vi "test-discretization-12-callback.vi"(9 "Y":T1, 10 "T":dbl, 11 "Variant":variant) -> (0 "Error":bool, 3 "output matrix":T1)   [LabVIEW 2019]
uses:
  <vilib>/Analysis/Matrix/Datatypes/RealMatrix.ctl
  <vilib>/Rock Robotics/WPI/ThirdParty/JAS_Junk/TrajLib/MatBuilder_Create.vi
  <vilib>/Rock Robotics/WPI/ThirdParty/JAS_Junk/TrajLib/Trajectory_Library.lvlib
  <vilib>/Analysis/Matrix/NI_Matrix.lvlib
  <vilib>/Analysis/Matrix/Numeric/Multiply/Multiply - RM,R.vi
  <vilib>/Analysis/NI_AALBase.lvlib
  <vilib>/Analysis/baseanly.llb/Real A x B.vi
panel:
  in  "Cluster":cluster{"ContQ":T1, "ContA":T1}
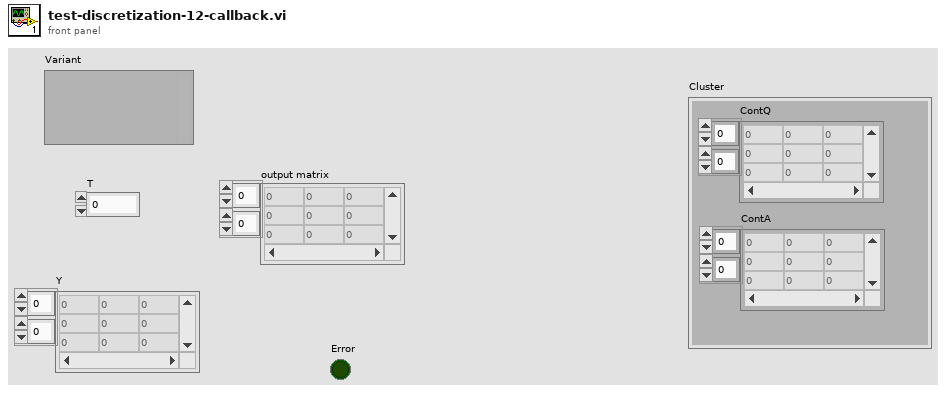
[diagram p1: front panel]
types:
  T1 = typedef "NI_Matrix.lvlib/RealMatrix.ctl" = dbl[][]
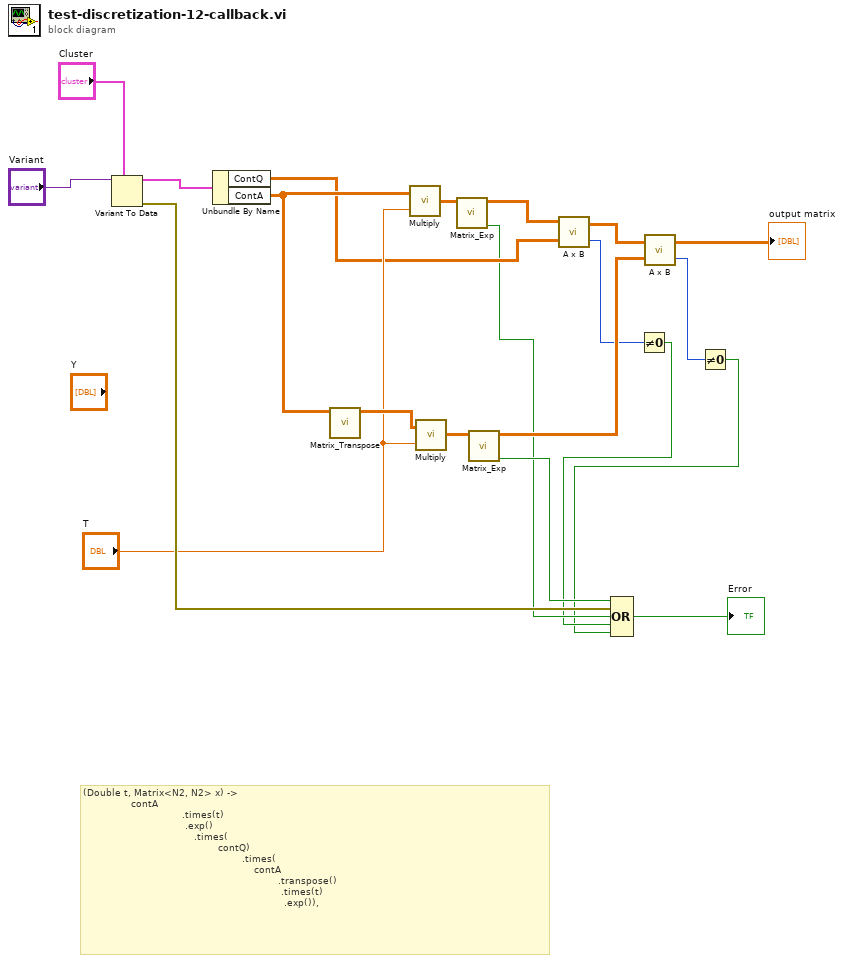
[diagram p0: block diagram]
diagram:
  # "(Double t, Matrix<N2, N2> x) ->\n                contA\n                                 .times(t)\n                                  .exp()\n                                     .times(  \n                                             contQ)\n                                                     .times(\n                                                         contA\n                                                                 .transpose()\n                                                                  .times(t)\n                                                                   .exp()),"
  n1 = Variant To Data(type="Cluster", Variant="Variant") -> (data=w18:cluster{"ContQ":T1, "ContA":T1}, error out=w15:errorcluster)  [unwired: 1 in]
  n2 = Unbundle By Name(w18) -> ("ContQ"=w10:T1, "ContA"=w14:T1)
  n3 = call <vilib>:"Matrix_Transpose.vi"("input matrix"=w14) -> ("output matrix"=w21:T1)  [unwired: 10 in]
  n4 = call-poly <vilib>:"Multiply.vi"("Real Scalar c"="T", "Real Matrix A"=w14) -> ("A * c"=w12:T1)
  n5 = call-poly <vilib>:"Multiply.vi"("Real Scalar c"="T", "Real Matrix A"=w21) -> ("A * c"=w17:T1)
  n6 = call <vilib>:"Matrix_Exp.vi"("input matrix"=w12) -> ("Error"=w6:bool, "output matrix"=w11:T1)  [unwired: 9 in]
  n7 = call <vilib>:"Matrix_Exp.vi"("input matrix"=w17) -> ("Error"=w16:bool, "output matrix"=w8:T1)  [unwired: 9 in]
  n8 = call-poly <vilib>:"A x B.vi"("B"=w10, "A"=w11) -> ("error"=w5:i32, "A x B"=w9:T1)
  n9 = Not Equal To 0?(x=w5) -> (x != 0?=w3:bool)
  n10 = call-poly <vilib>:"A x B.vi"("B"=w8, "A"=w9) -> ("error"=w4:i32, "A x B"=→"output matrix":T1)
  n11 = Not Equal To 0?(x=w4) -> (x != 0?=w2:bool)
  n12 = Compound Arithmetic op=OR(w16, w15, w6, w3, w2) -> (→"Error":bool)
